vi "MakeWall.vi"(7 "WallID":T1, 8 "error in (no error)":errorcluster, 11 "MazeGame":refnum<class "MazeGame.lvclass">) -> (0 "error out":errorcluster, 2 "Wall":refnum<class "Wall.lvclass">, 3 "MazeGame":refnum<class "MazeGame.lvclass">)   [LabVIEW 2020, in "FactoryMethod.lvlib" / "ParameterizedFactoryMethod.lvlib" / "MazeGame.lvclass"]
uses:
  MazeGame.lvclass
  GoFcommonClasses/ConcreteMazeSite/Wall/Wall.lvclass
  TypeDef/WallID.ctl
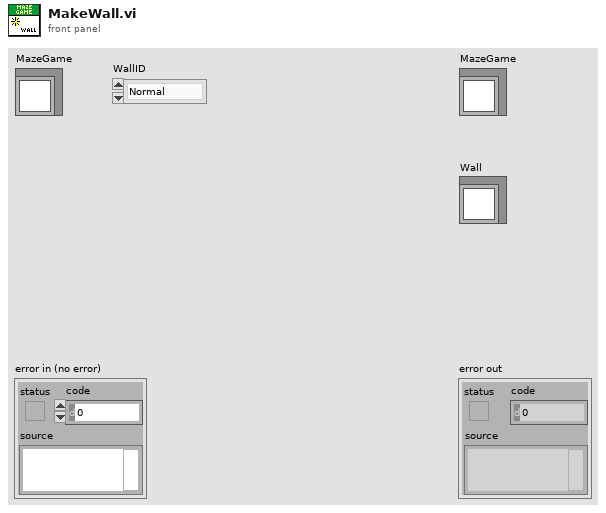
[diagram p1: front panel]
types:
  T1 = typedef "MazeGame.lvclass/WallID.ctl" = enum8{"Normal", "Bombed"}
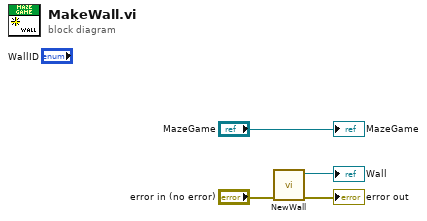
[diagram p0: block diagram]
diagram:
  n1 = call "NewWall.vi"("error in (no error)"="error in (no error)") -> ("error out"=→"error out":errorcluster, "Wall"=→"Wall":refnum<class "Wall.lvclass">)  [unwired: 9 in]
  "MazeGame" <- "MazeGame"
